vi "Str_to_Ch_dis_ADAM.vi"(4 "String Row":string) -> (0 "Value":dbl format="%.2f", 1 "Ch Description":T2={"Ch Name"="", "Type"="", "Function"=enum."Analogue Input", "Ch State"=enum."On", "Calibration type"="", "A"=0.0, "B"=0.0, "C"=0.0, "D"=0.0, "Comments"="", "Address"={"Main"=0, "Ch."=0, "Sub"=0, "Port Name"=""}, "String"="", "Duty"=65535} {"Duty" format="%016b"; "D" format="%#_5g"; "C" format="%#_5g"; "B" format="%#_5g"; "A" format="%#_5g"})   [LabVIEW 2016]
uses:
  ADAM Controls/Ch_description_ADAM.ctl
  ADAM Controls/Module_type_ADAM.ctl
  ADAM Controls/Function_ADAM.ctl
  ADAM Controls/Channel_State.ctl
  ADAM Controls/Calib_type_ADAM.ctl
  ADAM Controls/Address.ctl
panel:
  in  "Calibration type":T1
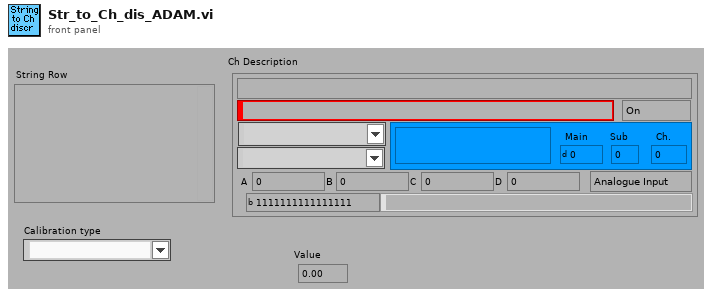
[diagram p1: front panel]
types:
  T1 = typedef "Calib_type_ADAM.ctl" = string
  T2 = typedef "Ch_description_ADAM.ctl" = cluster{"Ch Name":string, "Type":T3, "Function":T4, "Ch State":T5, "Calibration type":T1, "A":dbl, "B":dbl, "C":dbl, "D":dbl, "Comments":string, "Address":T6, "String":string, "Duty":u16}
  T3 = typedef "Module_type_ADAM.ctl" = string
  T4 = typedef "Function_ADAM.ctl" = enum16{"Analogue Input", "Digital Input", "Event counter", "Event rate", "Analogue Output", "Digital Output", "Relay Output"}
  T5 = typedef "Channel_State.ctl" = enum16{"On", "Off", "Always On", "Always Off"}
  T6 = typedef "Address.ctl" = cluster{"Main":i32, "Ch.":i32, "Sub":i32, "Port Name":string}
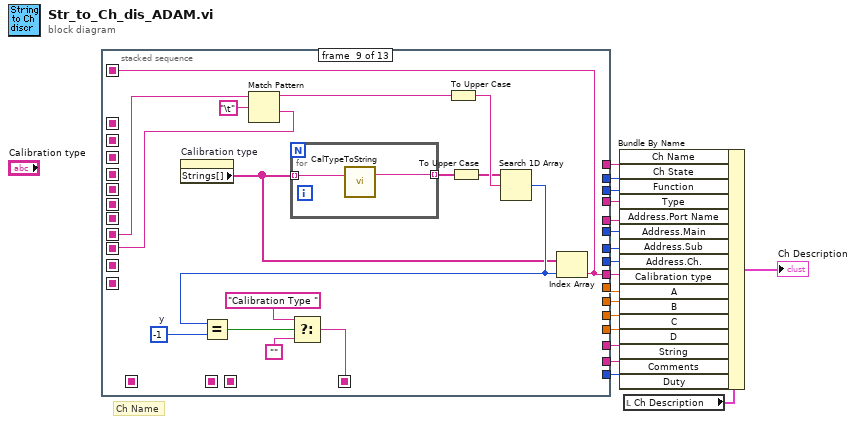
[diagram p0: block diagram]
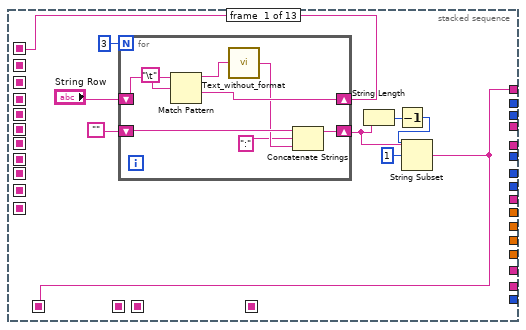
[diagram p2: hidden frame]
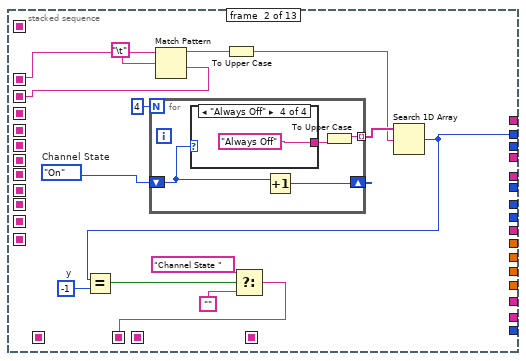
[diagram p3: hidden frame]
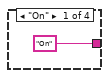
[diagram p4: hidden frame]
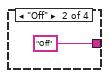
[diagram p5: hidden frame]
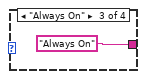
[diagram p6: hidden frame]
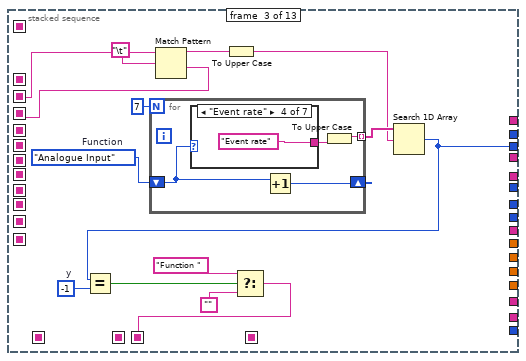
[diagram p7: hidden frame]
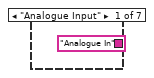
[diagram p8: hidden frame]
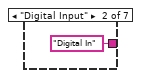
[diagram p9: hidden frame]
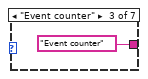
[diagram p10: hidden frame]
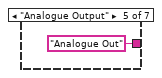
[diagram p11: hidden frame]
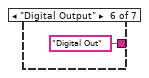
[diagram p12: hidden frame]
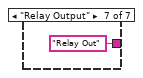
[diagram p13: hidden frame]
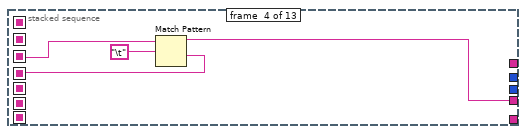
[diagram p14: hidden frame]
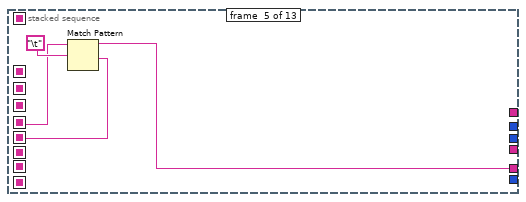
[diagram p15: hidden frame]
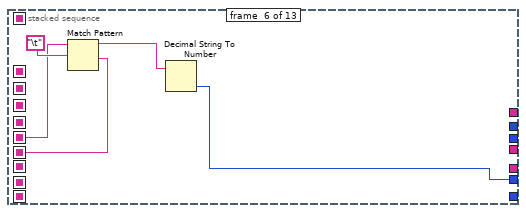
[diagram p16: hidden frame]
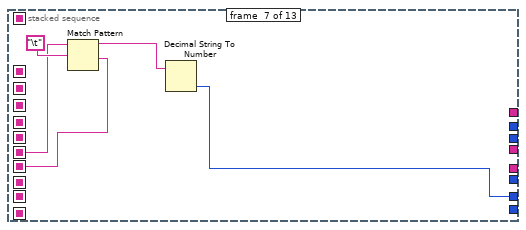
[diagram p17: hidden frame]
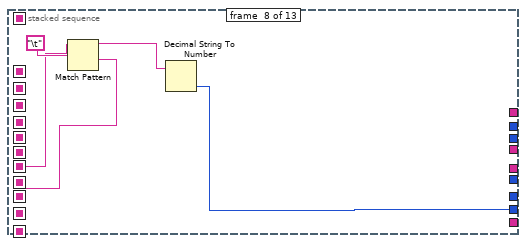
[diagram p18: hidden frame]
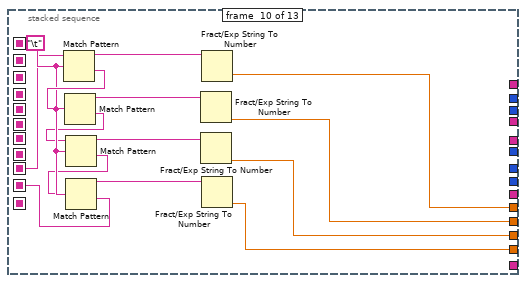
[diagram p19: hidden frame]
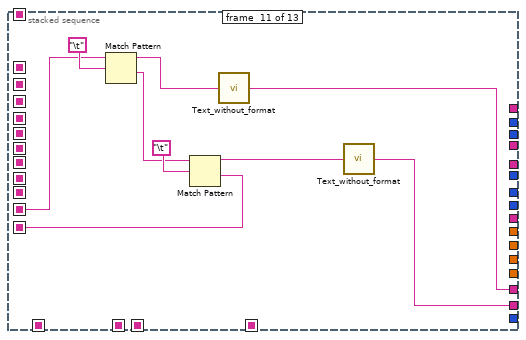
[diagram p20: hidden frame]
diagram:
  # "Ch Name"
  n1 = stacked-sequence {
    seq-local: [w24 _ _ _ _ _ _ _ _ _ _ _ _] -> [_ w43 _ _ _ _ _ _ _ _ _ _ _]
    seq-local: [_ w42 _ _ _ _ _ _ _ _ _ _ _] -> [_ _ w67 _ _ _ _ _ _ _ _ _ _]
    seq-local: [w19 _ _ _ _ _ _ _ _ _ _ _ _] -> [_ _ _ _ _ _ _ _ _ _ _ _ w156]
    seq-local: [_ _ w65 _ _ _ _ _ _ _ _ _ _] -> [_ _ _ w84 _ _ _ _ _ _ _ _ _]
    seq-local: [_ _ _ _ w89 _ _ _ _ _ _ _ _] -> [_ _ _ _ _ w93 _ _ _ _ _ _ _]
    seq-local: [_ _ _ _ _ _ _ w102 _ _ _ _ _] -> [_ _ _ _ _ _ _ _ w114 _ _ _ _]
    seq-local: [_ _ _ w85 _ _ _ _ _ _ _ _ _] -> [_ _ _ _ w88 _ _ _ _ _ _ _ _]
    seq-local: [_ _ _ _ _ _ _ _ _ w124 _ _ _] -> [_ _ _ _ _ _ _ _ _ _ w142 _ _]
    seq-local: [_ _ _ _ _ w92 _ _ _ _ _ _ _] -> [_ _ _ _ _ _ w98 _ _ _ _ _ _]
    seq-local: [_ _ _ _ _ _ w97 _ _ _ _ _ _] -> [_ _ _ _ _ _ _ w103 _ _ _ _ _]
    seq-local: [_ _ _ _ _ _ _ _ w113 _ _ _ _] -> [_ _ _ _ _ _ _ _ _ w123 _ _ _]
    seq-local: [_ _ _ _ _ _ _ _ _ _ w139 _ _] -> [_ _ _ _ _ _ _ _ _ _ _ w153 _]
    seq-local: [_ _ _ _ _ _ _ _ w111 _ _ _ _] -> [_ _ _ _ _ _ _ _ _ _ _ _ _]
    seq-local: [_ w36 _ _ _ _ _ _ _ _ _ _ _] -> [_ _ _ _ _ _ _ _ _ _ _ _ w160]
    seq-local: [_ _ w58 _ _ _ _ _ _ _ _ _ _] -> [_ _ _ _ _ _ _ _ _ _ _ _ w159]
    seq-local: [_ _ _ _ _ _ _ _ w107 _ _ _ _] -> [_ _ _ _ _ _ _ _ _ _ _ _ w155]
    tunnel: [_ _ w64 _ _ _ _ _ _ _ _ _ _] -> w18
    tunnel: [_ w40 _ _ _ _ _ _ _ _ _ _ _] -> w17
    tunnel: [_ _ _ _ w87 _ _ _ _ _ _ _ _] -> w14
    tunnel: [_ _ _ _ _ _ _ w101 _ _ _ _ _] -> w7
    tunnel: [_ _ _ _ _ _ _ _ w111 _ _ _ _] -> w8
    tunnel: [_ _ _ _ _ _ _ _ _ w136 _ _ _] -> w9
    tunnel: [_ _ _ _ _ _ _ _ _ w135 _ _ _] -> w10
    tunnel: [_ _ _ _ _ _ _ _ _ w134 _ _ _] -> w11
    tunnel: [_ _ _ _ _ _ _ _ _ w133 _ _ _] -> w12
    tunnel: [_ _ _ _ _ _ _ _ _ _ w143 _ _] -> w13
    tunnel: [w19 _ _ _ _ _ _ _ _ _ _ _ _] -> w15
    tunnel: [_ _ _ _ _ w91 _ _ _ _ _ _ _] -> w6
    tunnel: [_ _ _ _ _ _ w96 _ _ _ _ _ _] -> w5
    tunnel: [_ _ _ _ _ _ _ _ _ _ w137 _ _] -> w3
    tunnel: [_ _ _ _ _ _ _ _ _ _ _ w148 _] -> w2
    tunnel: [_ _ _ w83 _ _ _ _ _ _ _ _ _] -> w1
    frame #0 {
      n2 = for {
        N: 3 -> [_]
        shift-right: [w33] -> w24
        shift-left: "String Row" -> [w34]
        shift-right: [w30] -> w23
        shift-left: "" -> [w31]
        n3 = Match Pattern(string=w34, regular expression="\t") -> (before substring=w32:string, after substring=w33:string)  [unwired: 3 out]
        n4 = call "Text_without_format.vi"("Input string"=w32) -> ("Output string"=w29:string)
        n5 = Concatenate Strings(w31, ":" ("String without format char"), w29) -> (w30:string)
      }
      n6 = String Length(string=w23) -> (length=w22:i32)
      n7 = Decrement(x=w22) -> (x-1=w21:i32)
      n8 = String Subset(string=w23, offset (0)=1, length (rest)=w21) -> (substring=w19:string)
    }
    frame #1 {
      w41 = Channel_State."On"  # Channel State
      w46 = -1  # y
      n9 = for {
        N: 4 -> [_]
        shift-right: [w53] -> _
        shift-left: w41 -> [w51]
        tunnel: [w52] -> w48 mode=indexing
        n10 = case shown="\"Always Off\"" w51 {
          tunnel: ["On" "Off" "Always On" "Always Off"] -> w50
          frame "On" {
          }
          frame "Off" {
          }
          frame "Always On" {
          }
          frame "Always Off" {
          }
        }
        n11 = Increment(x=w51) -> (x+1=w53:T5)
        n12 = To Upper Case(1:w50) -> (0:w52:string)
      }
      n13 = Match Pattern(string=w43, regular expression="\t") -> (before substring=w45:string, after substring=w42:string)  [unwired: 3 out]
      n14 = To Upper Case(1:w45) -> (0:w44:string)
      n15 = Search 1D Array(1D array=w48, element=w44) -> (index of element=w40:i32)  [unwired: 1 out]
      n16 = Equal?(x=w40, y=w46) -> (x = y?=w37:bool)
      n17 = Select(t="Channel State ", s=w37, f="") -> (s? t:f=w36:string)
    }
    frame #2 {
      w62 = Function_ADAM."Analogue Input"  # Function
      w68 = -1  # y
      n18 = for {
        N: 7 -> [_]
        shift-right: [w75] -> _
        shift-left: w62 -> [w73]
        tunnel: [w74] -> w70 mode=indexing
        n19 = case shown="\"Event rate\"" w73 {
          tunnel: ["Analogue In" "Digital In" "Event counter" "Event rate" "Analogue Out" "Digital Out" "Relay Out"] -> w72
          frame "Analogue Input" {
          }
          frame "Digital Input" {
          }
          frame "Event counter" {
          }
          frame "Event rate" {
          }
          frame "Analogue Output" {
          }
          frame "Digital Output" {
          }
          frame "Relay Output" {
          }
        }
        n20 = Increment(x=w73) -> (x+1=w75:T4)
        n21 = To Upper Case(1:w72) -> (0:w74:string)
      }
      n22 = Match Pattern(string=w67, regular expression="\t") -> (before substring=w66:string, after substring=w65:string)  [unwired: 3 out]
      n23 = To Upper Case(1:w66) -> (0:w63:string)
      n24 = Search 1D Array(1D array=w70, element=w63) -> (index of element=w64:i32)  [unwired: 1 out]
      n25 = Equal?(x=w64, y=w68) -> (x = y?=w59:bool)
      n26 = Select(t="Function ", s=w59, f="") -> (s? t:f=w58:string)
    }
    frame #3 {
      n27 = Match Pattern(string=w84, regular expression="\t") -> (before substring=w83:string, after substring=w85:string)  [unwired: 3 out]
    }
    frame #4 {
      n28 = Match Pattern(string=w88, regular expression="\t") -> (before substring=w87:string, after substring=w89:string)  [unwired: 3 out]
    }
    frame #5 {
      n29 = Match Pattern(string=w93, regular expression="\t") -> (before substring=w94:string, after substring=w92:string)  [unwired: 3 out]
      n30 = Decimal String To Number(string=w94) -> (number=w91:i32)  [unwired: 3 out]
    }
    frame #6 {
      n31 = Match Pattern(string=w98, regular expression="\t") -> (before substring=w99:string, after substring=w97:string)  [unwired: 3 out]
      n32 = Decimal String To Number(string=w99) -> (number=w96:i32)  [unwired: 3 out]
    }
    frame #7 {
      n33 = Match Pattern(string=w103, regular expression="\t") -> (before substring=w104:string, after substring=w102:string)  [unwired: 3 out]
      n34 = Decimal String To Number(string=w104) -> (number=w101:i32)  [unwired: 3 out]
    }
    frame #8 {
      w118 = -1  # y
      n35 = property on="Calibration type" class="CmbBox (strict)"() -> ("Strings[]"=w106:string[])  [unwired: 2 in, 2 out]
      n36 = Match Pattern(string=w114, regular expression="\t") -> (before substring=w117:string, after substring=w113:string)  [unwired: 3 out]
      n37 = for {
        tunnel: [w121] -> w120 mode=indexing
        tunnel: w106 -> [w122] mode=indexing
        n38 = call "CalTypeToString.vi"("Calibration type"=w122) -> ("String"=w121:string)  [unwired: 2 in]
      }
      n39 = To Upper Case(1:w117) -> (0:w116:string)
      n40 = To Upper Case(1:w120) -> (0:w115:string[])
      n41 = Search 1D Array(1D array=w115, element=w116) -> (index of element=w112:i32)  [unwired: 1 out]
      n42 = Equal?(x=w112, y=w118) -> (x = y?=w108:bool)
      n43 = Select(t="Calibration Type ", s=w108, f="") -> (s? t:f=w107:string)
      n44 = Index Array(array=w106, index=w112) -> (element=w111:string)
    }
    frame #9 {
      w131 = "\t"
      n45 = Match Pattern(string=w123, regular expression=w131) -> (before substring=w128:string, after substring=w132:string)  [unwired: 3 out]
      n46 = Match Pattern(string=w132, regular expression=w131) -> (before substring=w127:string, after substring=w130:string)  [unwired: 3 out]
      n47 = Match Pattern(string=w130, regular expression=w131) -> (before substring=w126:string, after substring=w129:string)  [unwired: 3 out]
      n48 = Match Pattern(string=w129, regular expression=w131) -> (before substring=w125:string, after substring=w124:string)  [unwired: 3 out]
      n49 = Fract/Exp String To Number(string=w127) -> (number=w135:dbl)  [unwired: 4 out]
      n50 = Fract/Exp String To Number(string=w126) -> (number=w134:dbl)  [unwired: 4 out]
      n51 = Fract/Exp String To Number(string=w128) -> (number=w136:dbl)  [unwired: 4 out]
      n52 = Fract/Exp String To Number(string=w125) -> (number=w133:dbl)  [unwired: 4 out]
    }
    frame #10 {
      n53 = Match Pattern(string=w142, regular expression="\t") -> (before substring=w144:string, after substring=w140:string)  [unwired: 3 out]
      n54 = Match Pattern(string=w140, regular expression="\t") -> (before substring=w138:string, after substring=w139:string)  [unwired: 3 out]
      n55 = call "Text_without_format.vi"("Input string"=w144) -> ("Output string"=w143:string)
      n56 = call "Text_without_format.vi"("Input string"=w138) -> ("Output string"=w137:string)
    }
    frame #11 {
      n57 = Match Pattern(string=w153, regular expression="\t") -> (before substring=w146:string, after substring=w150:string)  [unwired: 3 out]
      n58 = Match Pattern(string=w150, regular expression="\t") -> (before substring=w147:string)  [unwired: 4 out]
      n59 = Fract/Exp String To Number(string=w147) -> (number=→"Value":dbl)  [unwired: 4 out]
      n60 = Decimal String To Number(string=w146) -> (number=w149:i32)  [unwired: 3 out]
      n61 = To Unsigned Word Integer(number=w149) -> (unsigned 16bit integer=w148:u16)
    }
    frame #12 {
      n62 = Concatenate Strings(w160, w159, w155) -> (w157:string)
      n63 = Empty String/Path?(string/path=w157) -> (empty?=w158:bool)
      n64 = case shown="True" w158 {
        tunnel: w157 -> [w167 _]
        tunnel: w156 -> [w165 _]
        frame False {
          w161 = TRUE  # Dialog Box
          n65 = Concatenate Strings(w167, "Invalid for ch named ", w165) -> (w164:string)
          n66 = Bundle By Name(cluster=errorcluster {"status"=FALSE, "code"=0, "source"=""} ("error in (no error)"), "status"=TRUE ("Bundle Element"), "source"=w164) -> (w162:errorcluster)
          n67 = call "EnFlo_Error_Handler.vi"("error in (no error)"=w162, "Dialog Box (T)"=w161) -> ()  [unwired: 1 in, 3 out]
        }
        frame True {
        }
      }
    }
  }
  n68 = local read "Ch Description"() -> (w16:T2)
  n69 = Bundle By Name(cluster=w16, "Ch Name"=w15, "Ch State"=w17, "Function"=w18, "Type"=w1, "Address.Port Name"=w14, "Address.Main"=w6, "Address.Sub"=w5, "Address.Ch."=w7, "Calibration type"=w8, "A"=w9, "B"=w10, "C"=w11, "D"=w12, "String"=w13, "Comments"=w3, "Duty"=w2) -> (→"Ch Description":T2)
